vi "Handle PM Groupe.vi"(0 "Stand in":refnum<class "Stand.lvclass">, 11 "error in (no error)":errorcluster) -> (4 "Stand out":refnum<class "Stand.lvclass">, 14 "dt PMG":u32, 15 "error out":errorcluster)   [LabVIEW 2019, in "Stand.lvclass"]
uses:
  Stand.lvclass
  Stand.lvclass/Stand.ctl
  Device_class/Device.lvclass/Device.ctl
  PM_Group_class/PM_Group.lvclass/PM_Group.ctl
  SV_Puplisher_class/SV_Publisher.lvclass/SV_Publisher.ctl
  AI_class/AI.lvclass/AI.ctl
  AnalogComparator_class/AnalogComparator.lvclass/AnalogComparator.ctl
  Engine_1DO_2DI_class/Engine_1DO_2DI.lvclass/Engine_1DO_2DI.ctl
  PM_Group_class/HandleCmd.vi
  PM_Group_class/private/Handle M12.vi
  PM_Group_class/private/Handle M24.vi
  PM_Group_class/HandleCmd.vi/0e91dc30-495c-4c1b-9970-a125a349d0cc.vi
  Device_class/GetConfigInterface.vi
  Device_class/GetSvPublisher.vi
  SV_Puplisher_class/Set SV.vi
  Device_class/GetMessageInterface.vi
  AI_class/Get_Values.vi
  Engine_1DO_2DI_class/TupnOn.vi
  Engine_1DO_2DI_class/GetEngineState.vi
  Device_class/GetFPGA.vi
  SV_Puplisher_class/Set SV.vi/1ae5d02c-efd0-450a-8aa4-8388e25d05bc.vi
  AnalogComparator_class/GetStatus.vi
  PM_Group_class/PM_Group.lvclass
  D:/GIT H4000/H4000/src/Device_class/Device.lvclass
  Engine_1DO_2DI_class/Engine_1DO_2DI.lvclass
  <vilib>/addons/_JKI.lib/Serialization/JSON/Library/Unflatten From JSON String.vi
  Engine_1DO_2DI_class/TupnOff.vi
  FPGA_API_class/Read Di.vi
  FPGA_API_class/Read DO.vi
  FPGA_API_class/Write Do.vi
  PM_Group_class/private/Handle M21.vi
  Engine_1DO_2DI_class/UpdateEngine.vi
  MessageInterface_class/MessageInterface.lvclass
  ConfigInterface_class/ConfigInterface.lvclass
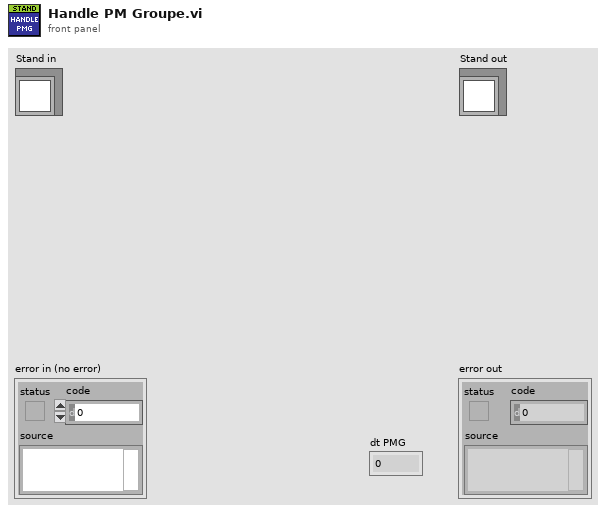
[diagram p1: front panel]
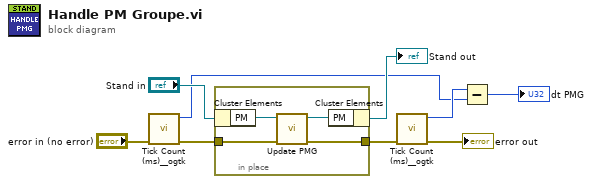
[diagram p0: block diagram]
diagram:
  n1 = call <userlib>:"Tick Count (ms)__ogtk.vi"("error in (no error)"="error in (no error)") -> ("error out"=w6:errorcluster, "millisecond timer value"=w2:u32)  [unwired: 9 in]
  n2 = in-place {
    in-place-border: w6 -> [w11]
    in-place-border: [w10] -> w5
    n3 = in-place-cluster #1("Stand in") -> ("PM"=w13:refnum<class "PM_Group.lvclass">)
    n4 = call "Update PMG.vi"("error in (no error)"=w11, "Pump_1AI_1DO_2DI in"=w13) -> ("error out"=w10:errorcluster, "Pump_1AI_1DO_2DI out"=w12:refnum<class "PM_Group.lvclass">)  [unwired: 8 in]
    n5 = in-place-cluster #1("PM"=w12) -> (→"Stand out":refnum<class "Stand.lvclass">)
  }
  n6 = call <userlib>:"Tick Count (ms)__ogtk.vi"("error in (no error)"=w5) -> ("error out"=→"error out":errorcluster, "millisecond timer value"=w3:u32)  [unwired: 9 in]
  n7 = Subtract(x=w3, y=w2) -> (x-y=→"dt PMG":u32)
